vi "GV_YscaleDataMinMax.vi"(5 "IncludeMinMax":bool, 6 "error in (no error)":errorcluster, 7 "Graph-ref":refnum<vi>, 8 "Plot":i32, 9 "Scale-min":dbl, 10 "Scale-max":dbl, 11 "PAQ-data":T1) -> (0 "min":dbl, 1 "Coord-min":i32, 2 "max":dbl, 3 "Coord-max":i32, 4 "error out":errorcluster)   [LabVIEW 2020, in "Sgraph_lib_V1.lvlib" / "Gviewer.lvclass"]
uses:
  Gviewer.lvclass
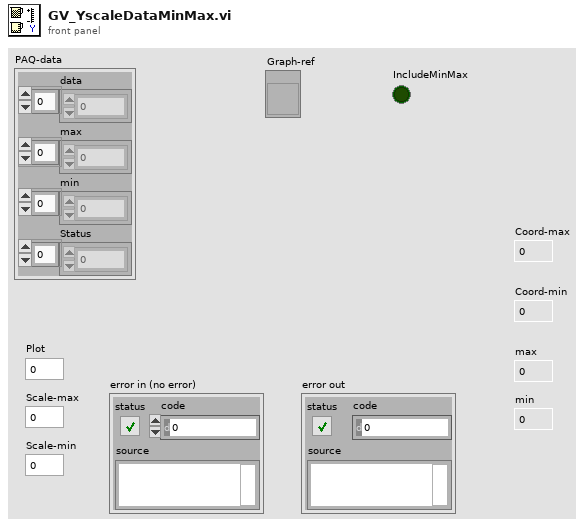
[diagram p1: front panel]
types:
  T1 = cluster{"data":dbl[], "max":dbl[], "min":dbl[], "Status":u32[]}
  T2 = typedef "LVRectTypeDef.ctl" = cluster{"Left":i16, "Top":i16, "Right":i16, "Bottom":i16}
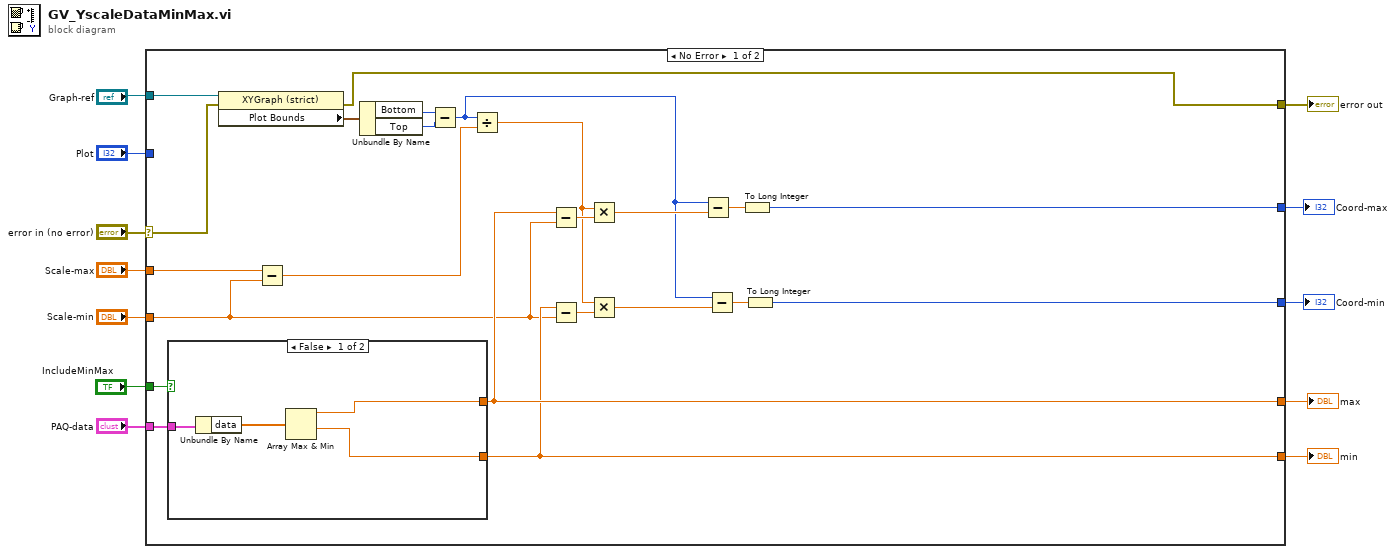
[diagram p0: block diagram]
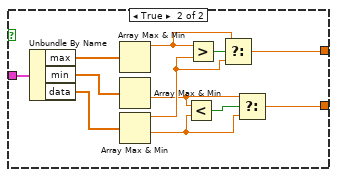
[diagram p2: hidden frame]
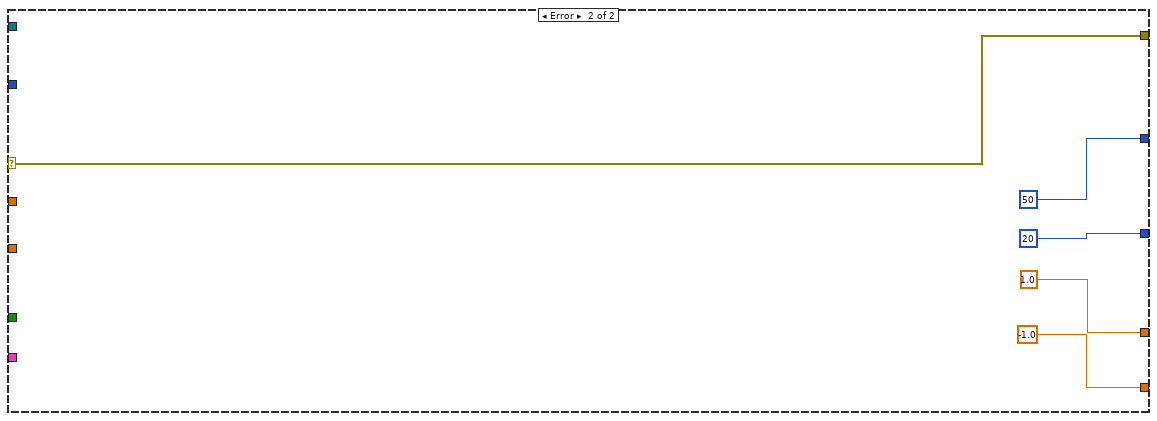
[diagram p3: hidden frame]
diagram:
  n1 = case shown="No Error" "error in (no error)" {
    selector: "error in (no error)" -> [w33 w56]
    tunnel: "PAQ-data" -> [w35 _]
    tunnel: "Plot" -> [_ _]
    tunnel: "Graph-ref" -> [w34 _]
    tunnel: [w27 1.0] -> w9
    tunnel: [w23 -1.0] -> w8
    tunnel: [w15 50 ("Vertical")] -> w2
    tunnel: [w14 20 ("Vertical")] -> w3
    tunnel: [w18 w56] -> w6
    tunnel: "Scale-max" -> [w29 _]
    tunnel: "Scale-min" -> [w22 _]
    tunnel: "IncludeMinMax" -> [w13 _]
    frame No Error {
      n2 = case shown="False" w13 {
        tunnel: w35 -> [w38 w51]
        tunnel: [w37 w41] -> w27
        tunnel: [w36 w40] -> w23
        frame False {
          n3 = Unbundle By Name(w38) -> ("data"=w39:dbl[])
          n4 = Array Max & Min(array=w39) -> (max value=w37:dbl, min value=w36:dbl)  [unwired: 2 out]
        }
        frame True {
          n5 = Unbundle By Name(w51) -> ("max"=w44:dbl[], "min"=w43:dbl[], "data"=w42:dbl[])
          n6 = Array Max & Min(array=w44) -> (max value=w49:dbl)  [unwired: 3 out]
          n7 = Array Max & Min(array=w43) -> (min value=w46:dbl)  [unwired: 3 out]
          n8 = Array Max & Min(array=w42) -> (max value=w48:dbl, min value=w45:dbl)  [unwired: 2 out]
          n9 = Less?(x=w46, y=w45) -> (x < y?=w47:bool)
          n10 = Greater?(x=w49, y=w48) -> (0:w50:bool)
          n11 = Select(t=w49, s=w50, f=w48) -> (s? t:f=w41:dbl)
          n12 = Select(t=w46, s=w47, f=w45) -> (s? t:f=w40:dbl)
        }
      }
      n13 = property class="XYGraph (strict)"(reference=w34, error in=w33) -> (error out=w18:errorcluster, "Plot Bounds"=w32:T2)  [unwired: 1 out]
      n14 = Subtract(x=w29, y=w22) -> (x-y=w28:dbl)
      n15 = Unbundle By Name(w32) -> ("Bottom"=w31:i16, "Top"=w30:i16)
      n16 = Subtract(x=w31, y=w30) -> (x-y=w20:i16)
      n17 = Divide(x=w20, y=w28) -> (x/y=w21:dbl)
      n18 = Subtract(x=w27, y=w22) -> (x-y=w26:dbl)
      n19 = Subtract(x=w23, y=w22) -> (x-y=w24:dbl)
      n20 = Multiply(x=w21, y=w26) -> (x*y=w25:dbl)
      n21 = Multiply(x=w21, y=w24) -> (x*y=w19:dbl)
      n22 = Subtract(x=w20, y=w25) -> (x-y=w17:dbl)
      n23 = Subtract(x=w20, y=w19) -> (x-y=w16:dbl)
      n24 = To Long Integer(number=w17) -> (32bit integer=w15:i32)
      n25 = To Long Integer(number=w16) -> (32bit integer=w14:i32)
    }
    frame Error {
    }
  }
  "max" <- w9
  "min" <- w8
  "Coord-min" <- w3
  "Coord-max" <- w2
  "error out" <- w6
